vi "Measurement Logic.vi"(8 "error in":errorcluster, 9 "measurement configuration":T2={"double in"=1.2, "Input Terminal Name"="", "DUT Pin"=""}, 10 "measure call context in":refnum<class "Measure Call Context.lvclass">) -> (0 "error out":errorcluster, 1 "measurement results":T1, 2 "measure call context out":refnum<class "Measure Call Context.lvclass">)   [LabVIEW 2025, in "Daqmx-Display.lvclass"]
doc: "Contains the core logic for executing the measurement."
uses:
  Daqmx-Display.lvclass
  <vilib>/Plug-In SDKs/Measurements/Measure Call Context/Measure Call Context.lvclass
  Measurement Configuration.ctl
  Measurement Results.ctl
  <vilib>/DAQmx/miscellaneous.llb/DAQmx Fill In Error Info.vi
  <extravilib>/ChannelInstances/Event Messenger-bool/Instantiate.vi
  Daqmx-Display.lvclass/Daqmx-Display.ctl
  <vilib>/DAQmx/create/channels.llb/DAQmx Create Channel (DI-Digital Input).vi
  <vilib>/DAQmx/read.llb/DAQmx Read (Digital 1D Bool 1Chan 1Samp).vi
  <vilib>/Plug-In SDKs/Clients/Session Management V1/Session Reservation/Session Reservation.lvclass
  session-management/daqmxDI/Session Management daqmxDI.lvlib
panel:
  out "stop":bool
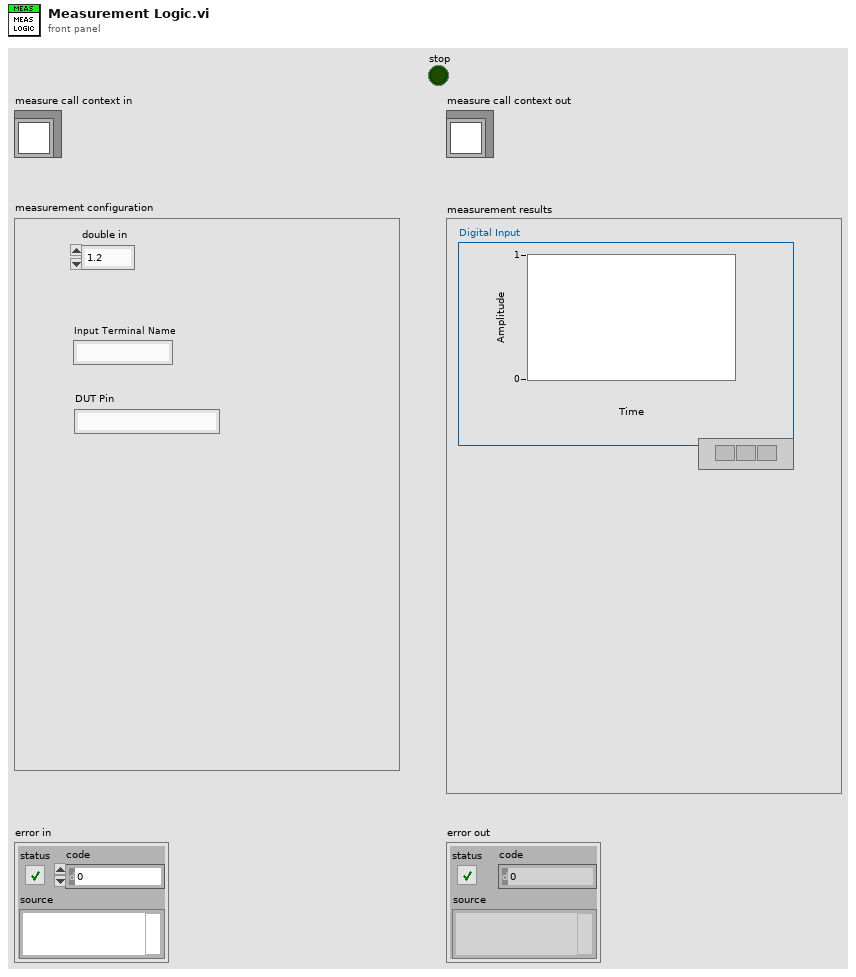
[diagram p1: front panel]
types:
  T1 = typedef "Daqmx-Display.lvclass/Measurement Results.ctl" = cluster{"Digital Input":u32[]}
  T2 = typedef "Daqmx-Display.lvclass/Measurement Configuration.ctl" = cluster{"double in":dbl, "Input Terminal Name":string, "DUT Pin":string}
  T3 = typedef "Event Messenger-bool.lvlib/))Channel.ctl" = refnum<queue>
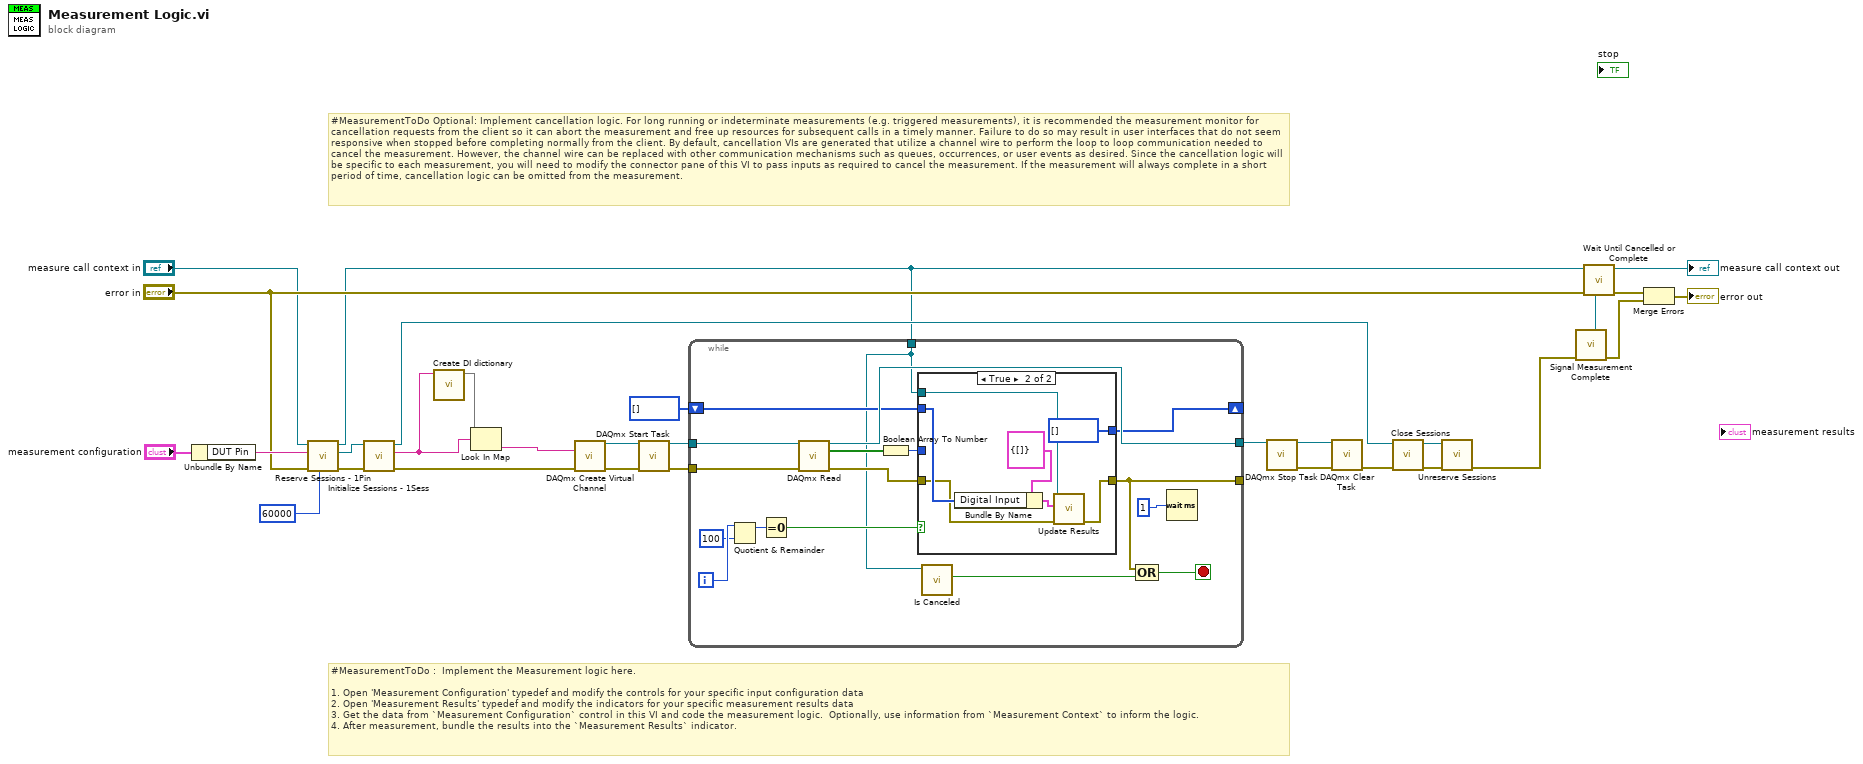
[diagram p0: block diagram]
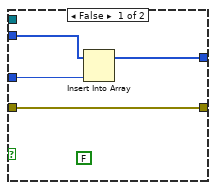
[diagram p2: hidden frame]
diagram:
  # "#MeasurementToDo Optional: Implement cancellation logic. For long running or indeterminate measurements (e.g. triggered measurements), it is recommended the measurement monitor for cancellation requests from the client so it can abort the measurement and free up resources for subsequent calls in a timely manner. Failure to do so may result in user interfaces that do not seem responsive when stopped before completing normally from the client. By default, cancellation VIs are generated that utilize a channel wire to perform the loop to loop communication needed to cancel the measurement. However, the channel wire can be replaced with other communication mechanisms such as queues, occurrences, or user events as desired. Since the cancellation logic will be specific to each measurement, you will need to modify the connector pane of this VI to pass inputs as required to cancel the measurement. If the measurement will always complete in a short period of time, cancellation logic can be omitted from the measurement."
  # "#MeasurementToDo :  Implement the Measurement logic here.\n\n1. Open 'Measurement Configuration' typedef and modify the controls for your specific input configuration data\n2. Open 'Measurement Results' typedef and modify the indicators for your specific measurement results data\n3. Get the data from `Measurement Configuration` control in this VI and code the measurement logic.  Optionally, use information from `Measurement Context` to inform the logic.\n4. After measurement, bundle the results into the `Measurement Results` indicator."
  n1 = Unbundle By Name("measurement configuration") -> ("DUT Pin"=w9:string)
  n2 = call <vilib>:"Reserve Sessions - 1Pin.vi"("timeout (ms)"=60000 ("timeout in milliseconds"), "error in"="error in", "pin or relay name"=w9, "measurement context in"="measure call context in") -> ("error out"=w7:errorcluster, "session reservation out"=w8:refnum<class "Session Reservation.lvclass">, "measurement context out"=w1:refnum<class "Measure Call Context.lvclass">)  [unwired: 5 in]
  n3 = call "Initialize Sessions - 1Sess.vi"("error in"=w7, "session reservation in"=w8) -> ("error out"=w4:errorcluster, "session"=w6:string, "session reservation out"=w3:refnum<class "Session Reservation.lvclass">)  [unwired: 6 in, 1 out]
  n4 = call "Create DI dictionary.vi"("PFI Input"=w6) -> ("map"=w17:map{string, string})  [unwired: 10 in]
  n5 = Look In Map(map=w17, key=w6) -> (value=w16:string)  [unwired: 1 in, 1 out]
  n6 = call-poly <vilib>:"DAQmx Create Virtual Channel.vi"("lines"=w16, "error in"=w4) -> ("task out"=w23:refnum<k21>, "error out"=w24:errorcluster)  [unwired: 12 in]
  n7 = call <vilib>:"DAQmx Start Task.vi"("task/channels in"=w23, "error in"=w24) -> ("task out"=w22:refnum<k21>, "error out"=w21:errorcluster)  [unwired: 12 in]
  n8 = while {
    tunnel: [w47] -> w18
    tunnel: w22 -> [w46]
    shift-right: [w38] -> _
    shift-left: u32[] [] -> [w37]
    tunnel: w21 -> [w35]
    tunnel: w1 -> [w32]
    tunnel: [w31] -> _
    i -> [w44]
    stop <- w36 stop-if-true
    n9 = Quotient & Remainder(x=w44, y=100) -> (x-y*floor(x/y)=w42:i32)  [unwired: 1 out]
    n10 = Equal To 0?(x=w42) -> (x = 0?=w41:bool)
    n11 = call-poly <vilib>:"DAQmx Read.vi"("task/channels in"=w46, "error in"=w35) -> ("task out"=w47:refnum<k21>, "data"=w40:bool[], "error out"=w34:errorcluster)  [unwired: 11 in]
    n12 = Boolean Array To Number(Boolean array=w40) -> (number=w39:u32)
    n13 = case shown="True" w41 {
      tunnel: w39 -> [w50 _]
      tunnel: w37 -> [w51 w56]
      tunnel: [w49 u32[] []] -> w38
      tunnel: w34 -> [w48 w53]
      tunnel: [w48 w52] -> w31
      tunnel: w32 -> [_ w55]
      frame False {
        (unwired) FALSE ("is canceled?")
        n14 = Insert Into Array(array=w51, new element=w50) -> (w49:u32[])  [unwired: 1 in]
      }
      frame True {
        n15 = Bundle By Name(cluster=T1 {"Digital Input"=[]} ("Measurement Results"), "Digital Input"=w56) -> (w54:T1)
        n16 = call <vilib>:"Update Results.vi"("error in"=w53, "measurement results"=w54, "measure call context in"=w55) -> ("error out"=w52:errorcluster)  [unwired: 7 in, 1 out]
      }
    }
    n17 = call <vilib>:"Is Canceled.vi"("measure call context in"=w32) -> ("is canceled?"=w33:bool)  [unwired: 8 in, 2 out]
    n18 = Compound Arithmetic op=OR(w31, w33) -> (w36:bool)
    n19 = Wait (ms)(milliseconds to wait=u32 1 ("Loop Time (ms)")) -> ()  [unwired: 1 out]
  }
  n20 = call <vilib>:"DAQmx Stop Task.vi"("task/channels in"=w18) -> ("task out"=w20:refnum<k21>, "error out"=w19:errorcluster)  [unwired: 13 in]
  n21 = call <vilib>:"DAQmx Clear Task.vi"("task in"=w20, "error in"=w19) -> ("error out"=w13:errorcluster)  [unwired: 13 in]
  n22 = call <vilib>:"Close Sessions.vi"("error in"=w13, "session reservation in"=w3) -> ("error out"=w12:errorcluster, "session reservation out"=w14:refnum<class "Session Reservation.lvclass">)  [unwired: 8 in]
  n23 = call <vilib>:"Unreserve Sessions.vi"("error in"=w12, "session reservation in"=w14) -> ("error out"=w11:errorcluster)  [unwired: 9 in]
  n24 = call "Signal Measurement Complete.vi"("error in (no error)"=w11) -> ("error out"=w28:errorcluster, "done channel"=w29:T3)  [unwired: 9 in]
  n25 = call "Wait Until Cancelled or Complete.vi"("done channel"=w29, "error in (no error)"="error in", "measure call context in"=w1) -> ("error out"=w27:errorcluster, "measure call context out"=→"measure call context out":refnum<class "Measure Call Context.lvclass">)  [unwired: 7 in]
  n26 = Merge Errors(w27, w28) -> (→"error out":errorcluster)
